vi "ADIS16448_RoboRIO_Teensy_FGV.vi"(6 "Reset":bool, 7 "Operation":enum16{"set", "get", "set reset"}(ring), 8 "error in":errorcluster, 9 "IMU AHRS":cluster{"Pitch":dbl, "Roll":dbl, "Yaw":dbl}, 10 "IMU Angles":T1, 11 "SerialPortRefIn":T2) -> (0 "error out":errorcluster, 1 "IMU AHRS Out":cluster{"Pitch":dbl, "Roll":dbl, "Yaw":dbl}, 2 "IMU Angles Out":T1, 3 "SerialPortRefOut":T2, 4 "Reset Out":bool)   [LabVIEW 2016, in "RoboRIO-Teensy-ADIS16448-Interface.lvlib"]
uses:
  RoboRIO-Teensy-ADIS16448-Interface.lvlib
  <vilib>/Rock Robotics/WPI/SerialPort/WPI_SerialPortRef.ctl
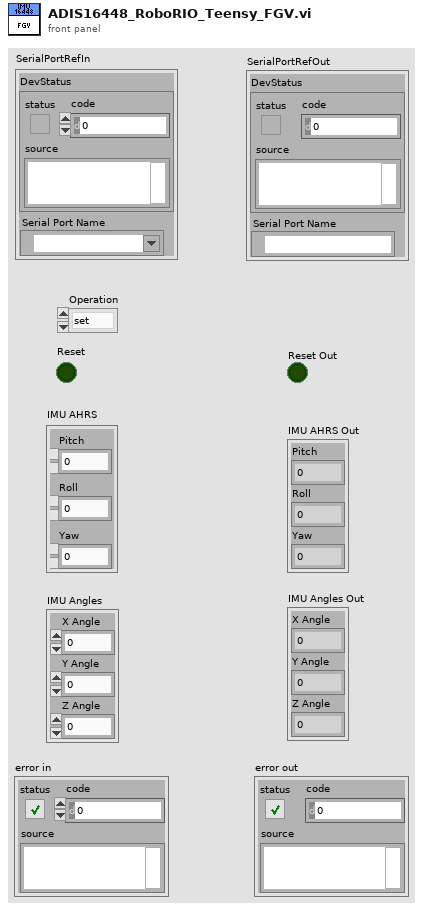
[diagram p1: front panel]
types:
  T1 = cluster{"X Angle":dbl, "Y Angle":dbl, "Z Angle":dbl}
  T2 = typedef "WPI_SerialPortRef.ctl" = cluster{"DevStatus":errorcluster, "Serial Port Name":refnum<visa-resource-name>}
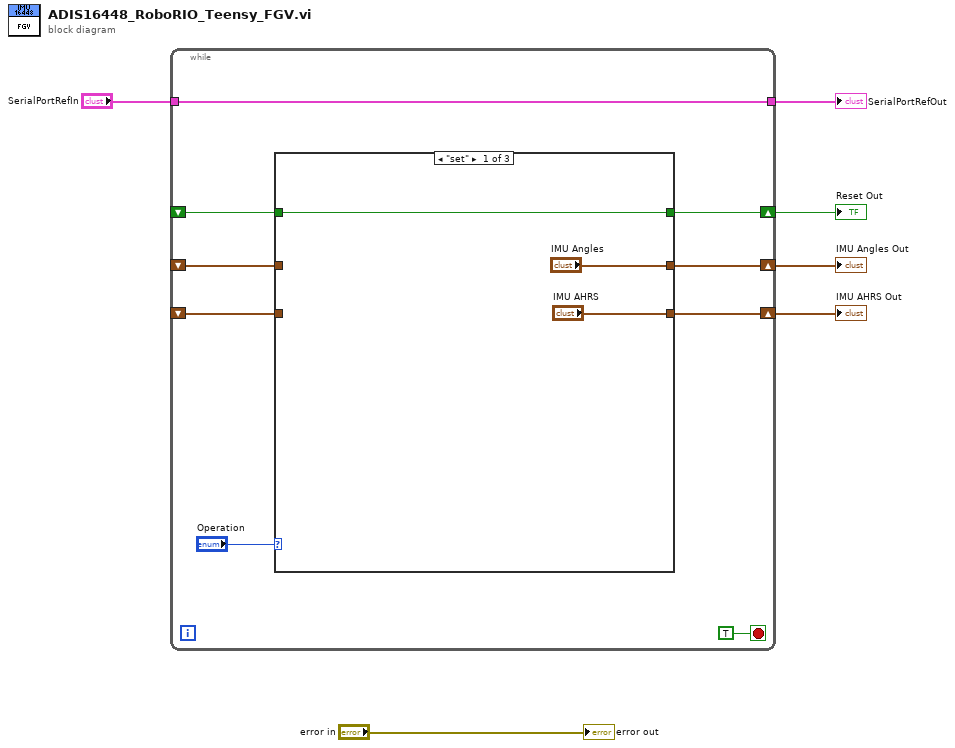
[diagram p0: block diagram]
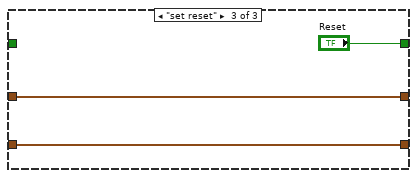
[diagram p3: hidden frame]
diagram:
  n1 = while {
    tunnel: [w14] -> w5
    tunnel: "SerialPortRefIn" -> [w14]
    shift-right: [w7] -> w2
    shift-left: _ -> [w8]
    shift-right: [w13] -> w4
    shift-left: _ -> [w12]
    shift-right: [w10] -> w3
    shift-left: _ -> [w9]
    stop <- TRUE stop-if-true
    n2 = case shown="\"set\"" "Operation" {
      tunnel: ["IMU Angles" w20 w23] -> w7
      tunnel: w8 -> [_ w20 w23]
      tunnel: ["IMU AHRS" w21 w22] -> w13
      tunnel: w12 -> [_ w21 w22]
      tunnel: w9 -> [w17 w19 _]
      tunnel: [w17 w19 "Reset"] -> w10
      frame "set" {
      }
      frame "get", Default {
      }
      frame "set reset" {
      }
    }
  }
  "SerialPortRefOut" <- w5
  "Reset Out" <- w3
  "IMU Angles Out" <- w2
  "IMU AHRS Out" <- w4
  "error out" <- "error in"
